vi "Init.vi"(8 "error in (no error)":errorcluster, 10 "Address":string, 11 "KeysightN9020B.lvlib:KeysightN9020B.lvclass":refnum<class "KeysightN9020B.lvclass">) -> (0 "error out":errorcluster, 3 "KeysightN9020B.lvlib:KeysightN9020B.lvclass":refnum<class "KeysightN9020B.lvclass">)   [LabVIEW 2023, in "KeysightN9020B.lvlib" / "KeysightN9020B.lvclass"]
uses:
  KeysightN9020B.lvclass
  typedefs/instrumentType.ctl
  KeysightN9020B.lvclass/KeysightN9020B.ctl
  <vilib>/ActorFramework/Actor/Actor.lvclass/Actor.ctl
  Interfaces/InitDeinitInterface/InitDeinitComm Messages/InitDone Msg/InitDone Msg.lvclass/InitDone Msg.ctl
  <vilib>/ActorFramework/Message Enqueuer/Message Enqueuer.lvclass/Message Enqueuer.ctl
  <vilib>/ActorFramework/Message Enqueuer/Enqueue.vi
  Interfaces/InitDeinitInterface/InitDeinitComm Messages/InitDone Msg/InitDone Msg.lvclass
  <vilib>/ActorFramework/Message Priority Queue/Priority Enqueue.vi
  <vilib>/ActorFramework/Actor/Actor.lvclass
  typedefs/typedefs.lvlib
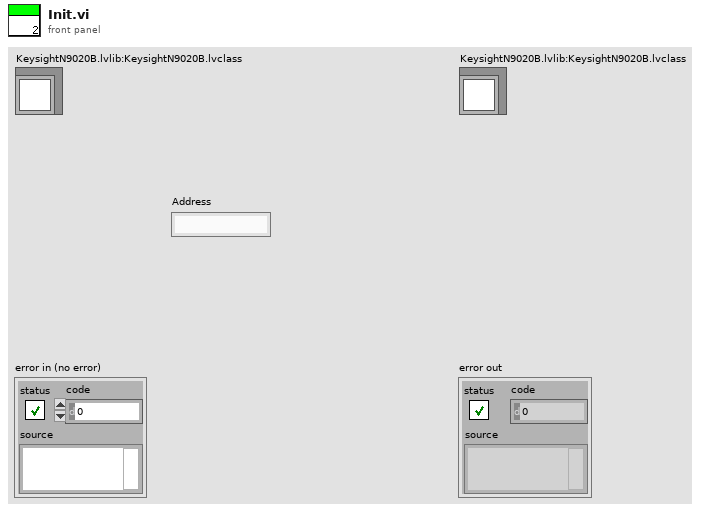
[diagram p1: front panel]
types:
  T1 = typedef "typedefs.lvlib/instrumentType.ctl" = enum16{"Spectrum Analyzer", "Spectrometer", "Camera", "Stepper", "Piezo", "SLM"}
  T2 = cluster{"address type":enum16{"VISA", "Index"}, "Address":string, "instrument type":T1}
  T3 = typedef "SpectrumAnalyzerData.ctl" = cluster{"Central Frequency":dbl, "Span":dbl}
  T4 = cluster{"Instr Error":errorcluster, "Spectrum Analyzer Data":T3, "Address":cluster{"address type":enum16{"VISA", "Index"}, "Address":string, "instrument type":T1}}
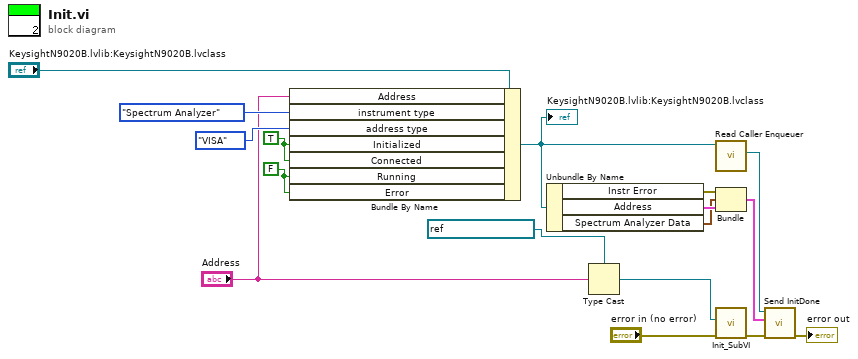
[diagram p0: block diagram]
diagram:
  w5 = FALSE ("InstrumentData.CurrentState.Running")
  w4 = TRUE ("InstrumentData.CurrentState.Running")
  n1 = Bundle By Name(cluster="KeysightN9020B.lvlib:KeysightN9020B.lvclass", "Address"="Address", "instrument type"=instrumentType."Spectrum Analyzer" ("InstrumentData.Address.instrument type"), "address type"=enum16{"VISA", "Index"}."VISA" ("InstrumentData.Address.address type"), "Initialized"=w4, "Connected"=w4, "Running"=w5, "Error"=w5) -> (w10:refnum<class "KeysightN9020B.lvclass">)
  "KeysightN9020B.lvlib:KeysightN9020B.lvclass" <- w10
  n2 = Unbundle By Name(w10) -> ("Instr Error"=w16:errorcluster, "Address"=w15:T2, "Spectrum Analyzer Data"=w14:T3)
  n3 = Type Cast(type=refnum<visa-resource-name> "Wave_Analyzer" ("Wave Analyzer"), x="Address") -> (*(type *) &x=w1:refnum<visa-resource-name>)
  n4 = call <vilib>:"Read Caller Enqueuer.vi"("Actor"=w10) -> ("Caller Enqueuer"=w7:refnum<class "Message Enqueuer.lvclass">)  [unwired: 10 in]
  n5 = Bundle("Instr Error"=w16, "Spectrum Analyzer Data"=w14, "Address"=w15) -> (w6:T4)  [unwired: 1 in]
  n6 = call "Init_SubVI.vi"("error in (no error)"="error in (no error)", "Wave Analyzer"=w1) -> ("error out"=w12:errorcluster)  [unwired: 9 in]
  n7 = call "Send InitDone.vi"("error in (no error)"=w12, "Variant"=w6, "Message Enqueuer"=w7) -> ("error out"=→"error out":errorcluster)  [unwired: 7 in, 1 out]
